vi "Split into 4.vi"(0 "Cx":dbl[](array[numeric]), 5 "Cy":dbl[](array[numeric]), 7 "Ix":dbl[](array[numeric]), 9 "Iy":dbl[](array[numeric])) -> (2 "C1x":dbl[](array[numeric]), 3 "C1y":dbl[](array[numeric]), 4 "C2x":dbl[](array[numeric]), 6 "C2y":dbl[](array[numeric]), 10 "C3x":dbl[](array[numeric]), 13 "C4x":dbl[](array[numeric]), 14 "C4y":dbl[](array[numeric]), 15 "C3y":dbl[](array[numeric]))   [LabVIEW 2023, in "d15.lvlib" / "Cave.lvclass"]
uses:
  Cave.lvclass
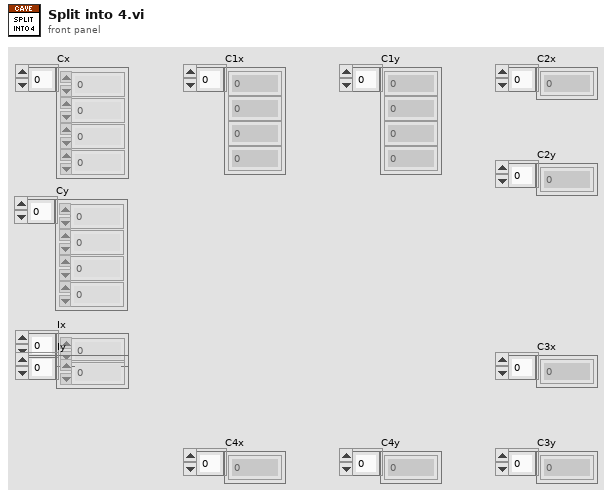
[diagram p1: front panel]
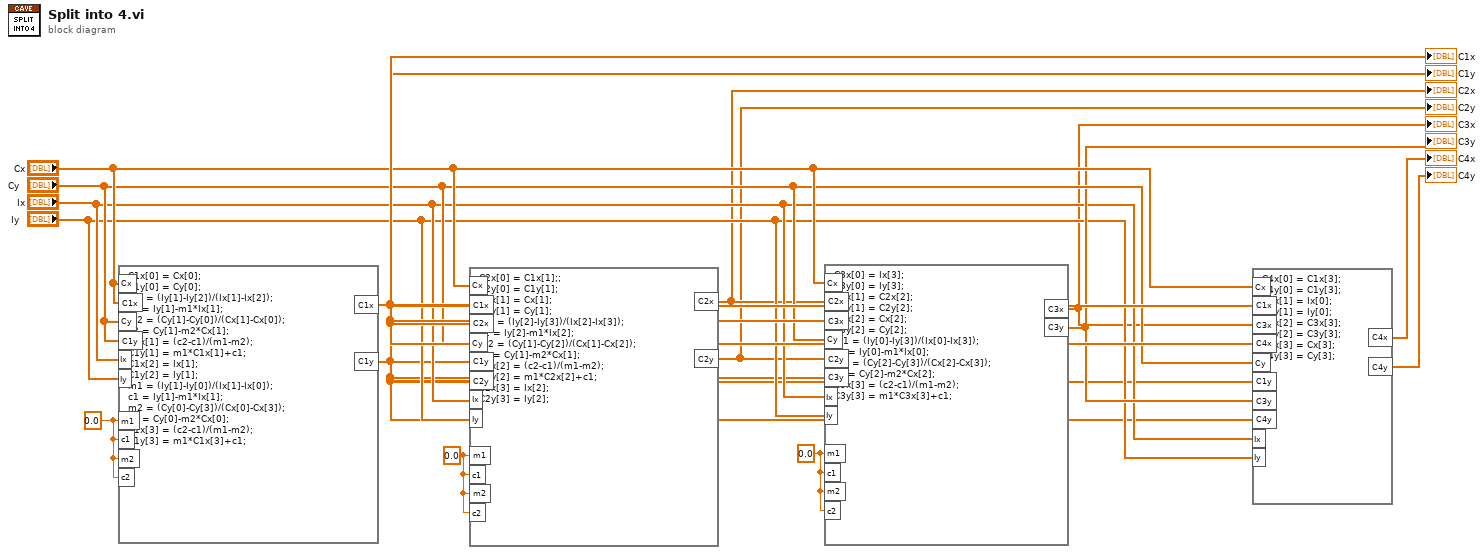
[diagram p0: block diagram]
diagram:
  w2 = 0.0 ("input variable")
  w5 = 0.0 ("input variable")
  w8 = 0.0 ("input variable")
  n1 = formula code="C1x[0] = Cx[0];\nC1y[0] = Cy[0];\nm1 = (Iy[1]-Iy[2])/(Ix[1]-Ix[2]);\nc1 = Iy[1]-m1*Ix[1];\nm2 = (Cy[1]-Cy[0])/(Cx[1]-Cx[0]);\nc2 = Cy[1]-m2*Cx[1];\nC1x[1] = (c2-c1)/(m1-m2);\nC1y[1] = m1*C1x[1]+c1;\nC1x[2] = Ix[1];\nC1y[2] = Iy[1];\nm1 = (Iy[1]-Iy[0])/(Ix[1]-Ix[0]);\nc1 = Iy[1]-m1*Ix[1];\nm2 = (Cy[0]-Cy[3])/(Cx[0]-Cx[3]);\nc2 = Cy[0]-m2*Cx[0];\nC1x[3] = (c2-c1)/(m1-m2);\nC1y[3] = m1*C1x[3]+c1;"("Cx"="Cx", "Ix"="Ix", "C1x"="Cx", "Cy"="Cy", "C1y"="Cy", "Iy"="Iy", "m1"=w8, "c1"=w8, "m2"=w8, "c2"=w8) -> ("C1x"=w15:dbl[], "C1y"=w1:dbl[])
  "C1x" <- w15
  "C1y" <- w1
  n2 = formula code="C2x[0] = C1x[1];;\nC2y[0] = C1y[1];\nC2x[1] = Cx[1];\nC2y[1] = Cy[1];\nm1 = (Iy[2]-Iy[3])/(Ix[2]-Ix[3]);\nc1 = Iy[2]-m1*Ix[2];\nm2 = (Cy[1]-Cy[2])/(Cx[1]-Cx[2]);\nc2 = Cy[1]-m2*Cx[1];\nC2x[2] = (c2-c1)/(m1-m2);\nC2y[2] = m1*C2x[2]+c1;\nC2x[3] = Ix[2];\nC2y[3] = Iy[2];"("Cx"="Cx", "Ix"="Ix", "C1x"=w15, "C2x"=w15, "Cy"="Cy", "C1y"=w1, "Iy"="Iy", "C2y"=w1, "m1"=w5, "c1"=w5, "m2"=w5, "c2"=w5) -> ("C2x"=w4:dbl[], "C2y"=w3:dbl[])
  "C2x" <- w4
  "C2y" <- w3
  n3 = formula code="C3x[0] = Ix[3];\nC3y[0] = Iy[3];\nC3x[1] = C2x[2];\nC3y[1] = C2y[2];\nC3x[2] = Cx[2];\nC3y[2] = Cy[2];\nm1 = (Iy[0]-Iy[3])/(Ix[0]-Ix[3]);\nc1 = Iy[0]-m1*Ix[0];\nm2 = (Cy[2]-Cy[3])/(Cx[2]-Cx[3]);\nc2 = Cy[2]-m2*Cx[2];\nC3x[3] = (c2-c1)/(m1-m2);\nC3y[3] = m1*C3x[3]+c1;"("Cx"="Cx", "Ix"="Ix", "C3x"=w15, "Cy"="Cy", "C3y"=w1, "Iy"="Iy", "C2x"=w4, "C2y"=w3, "m1"=w2, "c1"=w2, "m2"=w2, "c2"=w2) -> ("C3x"=w7:dbl[], "C3y"=w12:dbl[])
  "C3x" <- w7
  "C3y" <- w12
  n4 = formula code="C4x[0] = C1x[3];\nC4y[0] = C1y[3];\nC4x[1] = Ix[0];\nC4y[1] = Iy[0];\nC4x[2] = C3x[3];\nC4y[2] = C3y[3];\nC4x[3] = Cx[3];\nC4y[3] = Cy[3];"("Cx"="Cx", "Ix"="Ix", "C1x"=w15, "C3x"=w7, "C4x"=w15, "Cy"="Cy", "C1y"=w1, "C3y"=w12, "C4y"=w1, "Iy"="Iy") -> ("C4x"=→"C4x":dbl[], "C4y"=→"C4y":dbl[])
